vi "WriteData.vi"(8 "error in (no error)":errorcluster, 10 "Data":i16[][](array[numeric]), 11 "RFSoC Driver in":refnum<class "RFSoC Driver.lvclass">) -> (0 "error out":errorcluster, 2 "Responce out":string, 3 "RFSoC Driver out":refnum<class "RFSoC Driver.lvclass">)   [LabVIEW 2019, in "RFSoC Driver.lvclass"]
uses:
  RFSoC Driver.lvclass
  C:/github/NHMFL_Core/Libraries/Instruments/RFSoC/2019/GitHub/NHMFL_Core/Libraries/Instruments/Pulse Driver/Pulse Driver.lvclass
  Pulse Driver/Pulse Driver.lvclass/Pulse Driver.ctl
  RFSoC Driver.lvclass/RFSoC Driver.ctl
  Pulse Driver/Read Samples per read.vi
  Read Mixer.vi
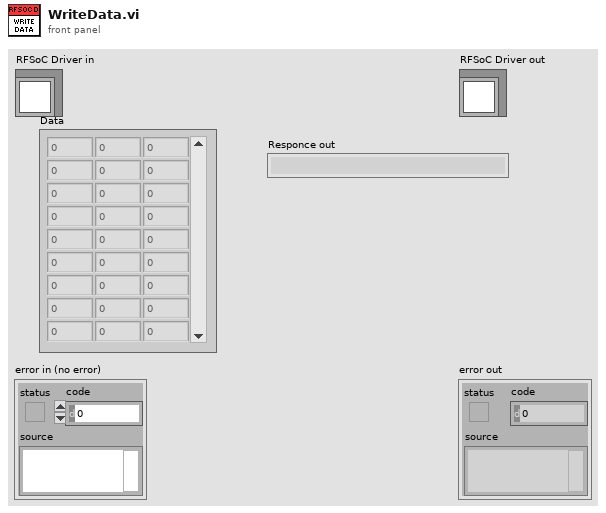
[diagram p1: front panel]
types:
  T1 = enum16{"Standard", "Buffered", "CRLF", "Immediate"}
  T2 = enum16{"big-endian, network order", "native, host order", "little-endian"}
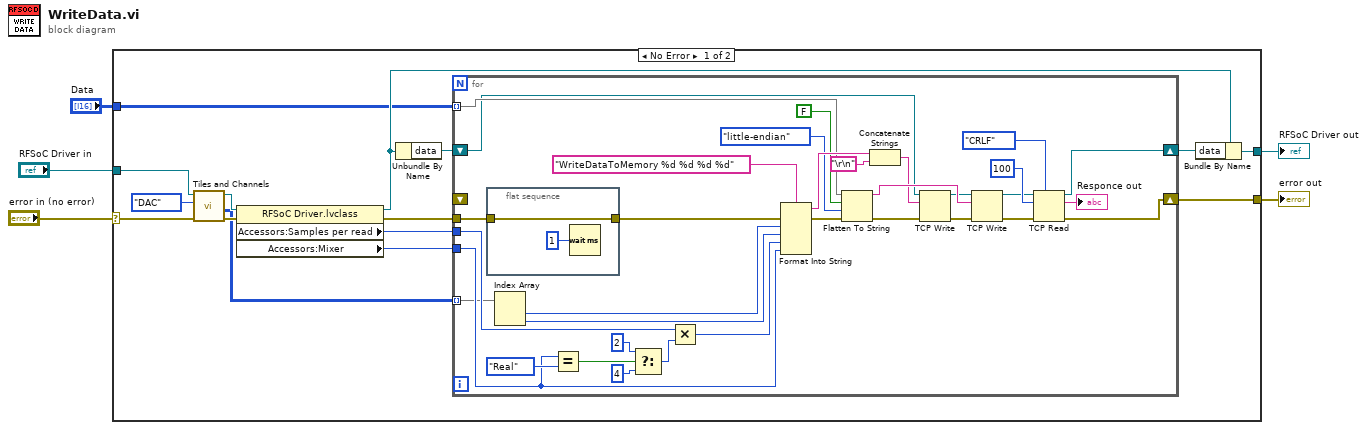
[diagram p0: block diagram]
diagram:
  n1 = case shown="No Error" "error in (no error)" {
    selector: "error in (no error)" -> [w10 w57]
    tunnel: [w20 w57] -> w4
    tunnel: [w13 w56] -> w2
    tunnel: "RFSoC Driver in" -> [w12 w56]
    tunnel: "Data" -> [w6 _]
    frame No Error {
      n2 = call-dynamic "Tiles and Channels.vi"("error in (no error)"=w10, "Type"=enum16{"ADC", "DAC"}."DAC", "RFSoC Driver in"=w12) -> ("error out"=w8:errorcluster, "Tiles and converters out"=w7:i32[][], "RFSoC Driver out"=w11:refnum<class "RFSoC Driver.lvclass">)  [unwired: 5 in, 1 out]
      n3 = property class="RFSoC Driver.lvclass"(reference=w11, error in=w8) -> (reference out=w16:refnum<class "RFSoC Driver.lvclass">, error out=w19:errorcluster, "Accessors:Samples per read"=w18:i32, "Accessors:Mixer"=w17:enum16{"Real", "I/Q"})
      n4 = Unbundle By Name(w16) -> ("data"=w15:refnum<k5>)
      n5 = for {
        shift-right: [w27] -> w20
        shift-left: _ -> [_]
        tunnel: w19 -> [w43]
        tunnel: w18 -> [w42]
        tunnel: w17 -> [w41]
        tunnel: w7 -> [w40] mode=indexing
        tunnel: w6 -> [w25] mode=indexing
        shift-right: [w22] -> w14
        shift-left: w15 -> [w24]
        n6 = flat-sequence {
          tunnel: [w54] -> w45
          tunnel: w43 -> [w54]
          frame #0 {
            n7 = Wait (ms)(milliseconds to wait=u32 1) -> ()  [unwired: 1 out]
          }
        }
        n8 = Index Array(array=w40) -> (element #1=w39:i32, element #2=w38:i32)  [unwired: 2 in]
        n9 = Equal?(x=w41, y=enum16{"Real", "I/Q"}."Real" ("Mixer")) -> (x = y?=w51:bool)
        n10 = Select(t=2 ("Binary sample width"), s=w51, f=4 ("Binary sample width")) -> (s? t:f=w47:i32)
        n11 = Multiply(x=w42, y=w47) -> (x*y=w44:i32)
        n12 = Format Into String(format string="WriteDataToMemory %d %d %d %d", error in=w45, w39, w38, w44, w41) -> (resulting string=w46:string, error out=w26:errorcluster)  [unwired: 1 in]
        n13 = Flatten To String(anything=w25, prepend array or string size? (T)=FALSE, byte order (0:big-endian, network order)=T2."little-endian", error in (no error)=w26) -> (data string=w33:string, error out=w30:errorcluster)  [unwired: 1 out]
        n14 = Concatenate Strings(w46, "\r\n") -> (w23:string)
        n15 = TCP Write(connection ID=w24, data in=w23, error in (no error)=w30) -> (connection ID out=w32:refnum<k5>, error out=w31:errorcluster)  [unwired: 1 in, 1 out]
        n16 = TCP Write(connection ID=w32, data in=w33, error in (no error)=w31) -> (connection ID out=w34:refnum<k5>, error out=w35:errorcluster)  [unwired: 1 in, 1 out]
        n17 = TCP Read(connection ID=w34, bytes to read=100, error in (no error)=w35, 7:T1."CRLF" ("mode (standard)")) -> (connection ID out=w22:refnum<k5>, data out=→"Responce out":string, error out=w27:errorcluster)  [unwired: 1 in]
      }
      n18 = Bundle By Name(cluster=w16, "data"=w14) -> (w13:refnum<class "RFSoC Driver.lvclass">)
    }
    frame Error {
    }
  }
  "error out" <- w4
  "RFSoC Driver out" <- w2
